vi "Show VI States.vi"() -> ()   [LabVIEW 2013]
panel:
  out "size":i32
  out "VI States":T1(array[cluster])
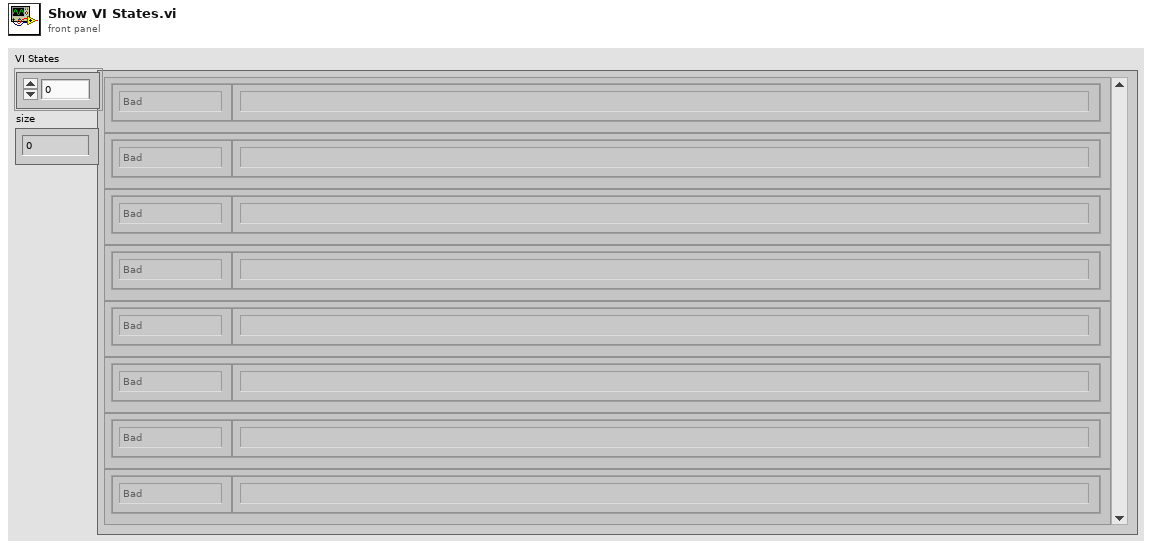
[diagram p1: front panel]
types:
  T1 = cluster{"Exec.State":enum32{"Bad", "Idle", "Run top level", "Running"}, "String":string}[]
  T2 = enum32{"Bad", "Idle", "Run top level", "Running"}
  T3 = cluster{"Exec.State":enum32{"Bad", "Idle", "Run top level", "Running"}, string}
  T4 = cluster{"Exec.State":enum32{"Bad", "Idle", "Run top level", "Running"}, string}[]
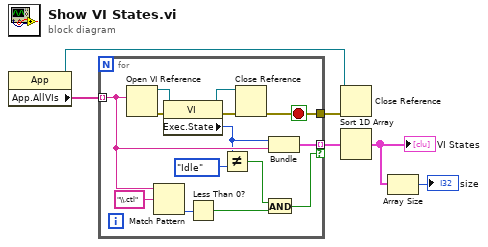
[diagram p0: block diagram]
diagram:
  n1 = property class="App"() -> (reference out=w5:refnum<vi>, "App.AllVIs"=w6:string[])  [unwired: 2 in, 1 out]
  n2 = for {
    tunnel: w6 -> [w14] mode=indexing
    tunnel: [w16] -> w4
    tunnel: [w15] -> w3 mode=indexing if=w10
    stop <- w16 stop-if-true
    n3 = Open VI Reference(vi path=w14) -> (vi reference=w19:refnum<vi>, error out=w20:errorcluster)  [unwired: 5 in]
    n4 = Match Pattern(string=w14, regular expression="\\.ctl") -> (offset past match=w12:i32)  [unwired: 1 in, 3 out]
    n5 = property class="VI"(reference=w19, error in=w20) -> (reference out=w18:refnum<vi>, error out=w17:errorcluster, "Exec.State"=w9:T2)
    n6 = Less Than 0?(x=w12) -> (x < 0?=w11:bool)
    n7 = Not Equal?(x=w9, y=T2."Idle" ("Execution:State")) -> (x != y?=w7:bool)
    n8 = Close Reference(reference=w18, error in (no error)=w17) -> (error out=w16:errorcluster)
    n9 = And(x=w7, y=w11) -> (x .and. y?=w10:bool)
    n10 = Bundle("Exec.State"=w9, w14) -> (w15:T3)  [unwired: 1 in]
  }
  n11 = Close Reference(reference=w5, error in (no error)=w4) -> ()  [unwired: 1 out]
  n12 = Sort 1D Array(array=w3) -> (sorted array=w2:T4)
  "VI States" <- w2
  n13 = Array Size(array=w2) -> (size(s)=→"size":i32)
